vi "TestExec.Msg to Result, Float.vi"(8 "error in":errorcluster, 11 "Msg":string[](array[string])) -> (0 "error out":errorcluster, 3 "Result":T1)   [LabVIEW 2016]
uses:
  Controls/TestExec.Comparison Enum.ctl
  Controls/TestExec.Result Cluster, Float.ctl
panel:
  in  "Limits":variant
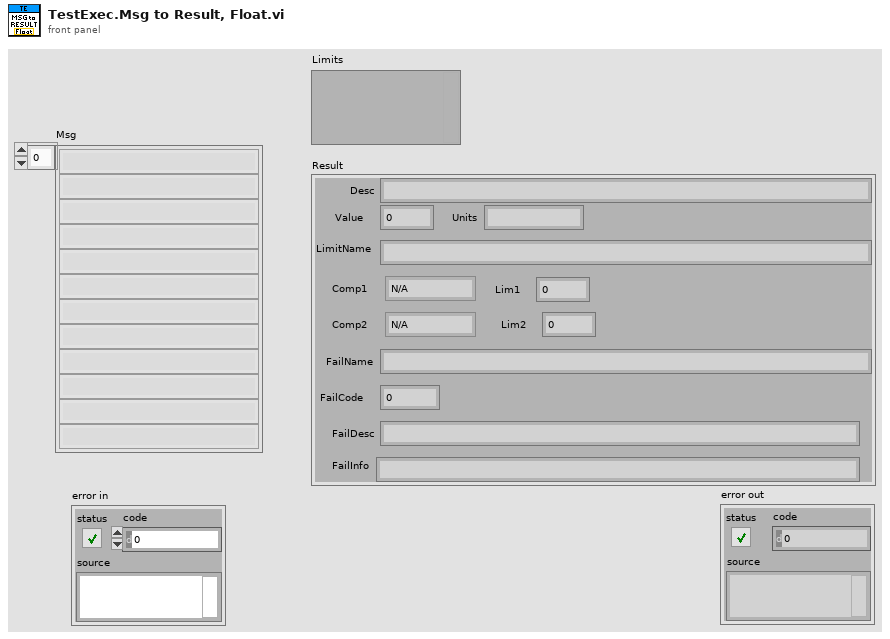
[diagram p1: front panel]
types:
  T1 = typedef "TestExec.Result Cluster, Float.ctl" = cluster{"Desc":string, "Value":dbl, "Units":string, "LimitName":string, "Comp1":T2, "Lim1":dbl, "Comp2":T2, "Lim2":dbl, "FailName":string, "FailCode":dbl, "FailDesc":string, "FailInfo":string}
  T2 = typedef "TestExec.Comparison Enum.ctl" = enum16{"N/A", "EQ", "NEQ", "LT", "LTE", "GT", "GTE"}
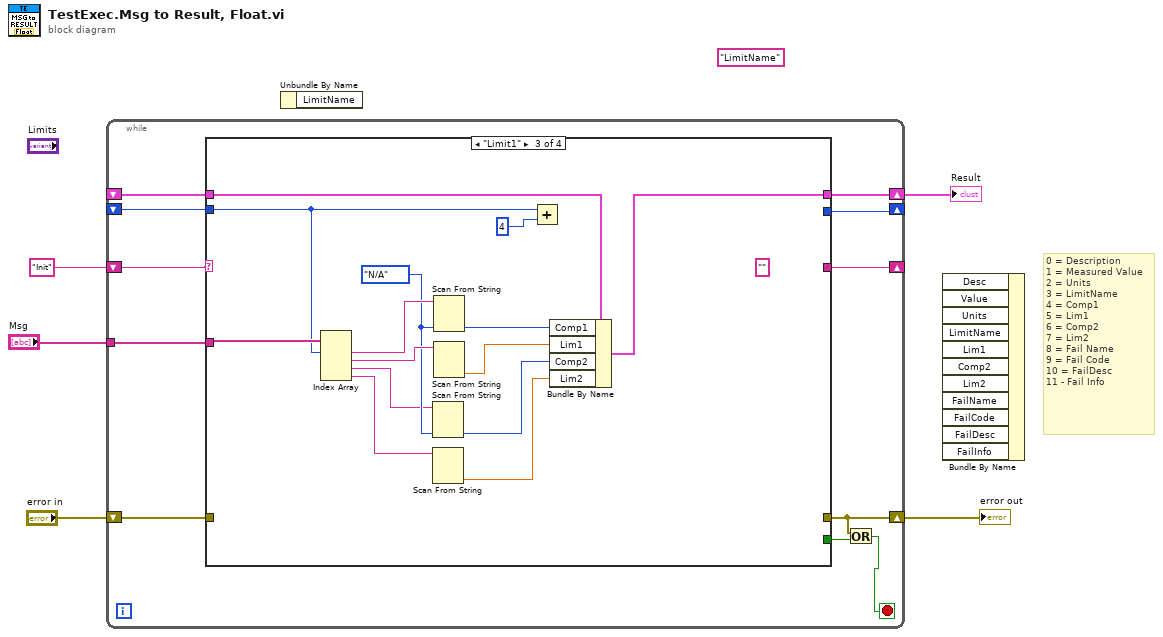
[diagram p0: block diagram]
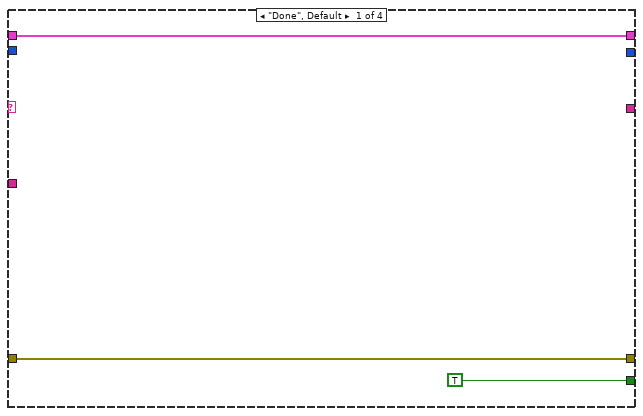
[diagram p2: hidden frame]
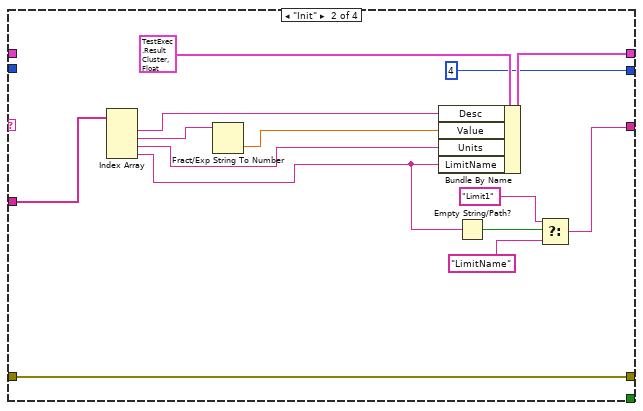
[diagram p3: hidden frame]
diagram:
  (unwired) "LimitName"
  # "0 = Description\t\n1 = Measured Value \n2 = Units\n3 = LimitName\t\n4 = Comp1\t\t\n5 = Lim1 \t\n6 = Comp2 \t\t\n7 = Lim2 \t\n8 = Fail Name\n9 = Fail Code\n10 = FailDesc\n11 - Fail Info"
  n1 = while {
    tunnel: "Msg" -> [w12]
    shift-right: [w13] -> _
    shift-left: "Init" -> [w14]
    shift-right: [w15] -> w3
    shift-left: _ -> [w16]
    shift-right: [w9] -> w1
    shift-left: "error in" -> [w11]
    shift-right: [w6] -> _
    shift-left: _ -> [w7]
    stop <- w8 stop-if-true
    n2 = case shown="\"Limit1\"" w14 {
      tunnel: w16 -> [w17 _ w47 _]
      tunnel: [w17 w32 w36 _] -> w15
      tunnel: [_ w23 _ _] -> w13
      tunnel: w12 -> [_ w31 w46 _]
      tunnel: w11 -> [w18 w26 _ _]
      tunnel: [w18 w26 _ _] -> w9
      tunnel: [TRUE _ _ _] -> w10
      tunnel: w7 -> [_ _ w35 _]
      tunnel: [_ 4 _ _] -> w6
      frame "Done", Default {
      }
      frame "Init" {
        n3 = Index Array(array=w31) -> (element #1=w30:string, element #2=w28:string, element #3=w27:string, element #4=w21:string)  [unwired: 4 in]
        n4 = Fract/Exp String To Number(string=w28) -> (number=w29:dbl)  [unwired: 3 in, 1 out]
        n5 = Bundle By Name(cluster=T1 {"Desc"="", "Value"=0.0, "Units"="", "LimitName"="", "Comp1"=enum."N/A", "Lim1"=0.0, "Comp2"=enum."N/A", "Lim2"=0.0, "FailName"="", "FailCode"=0.0, "FailDesc"="", "FailInfo"=""} ("Result"), "Desc"=w30, "Value"=w29, "Units"=w27, "LimitName"=w21) -> (w32:T1)
        n6 = Empty String/Path?(string/path=w21) -> (empty?=w20:bool)
        n7 = Select(t="Limit1", s=w20, f="LimitName") -> (s? t:f=w23:string)
      }
      frame "Limit1" {
        w39 = TestExec.Comparison_Enum."N/A" ("Comp1")
        (unwired) ""
        n8 = Index Array(array=w46, index #1=w35) -> (element #1=w45:string, element #2=w42:string, element #3=w38:string, element #4=w37:string)  [unwired: 3 in]
        n9 = Scan From String(input string=w38, default 1=w39) -> (output 1=w41:T2)  [unwired: 3 in, 3 out]
        n10 = Scan From String(input string=w37) -> (output 1=w40:dbl)  [unwired: 4 in, 3 out]
        n11 = Scan From String(input string=w45, default 1=w39) -> (output 1=w44:T2)  [unwired: 3 in, 3 out]
        n12 = Scan From String(input string=w42) -> (output 1=w43:dbl)  [unwired: 4 in, 3 out]
        n13 = Add(x=w35, y=4) -> ()  [unwired: 1 out]
        n14 = Bundle By Name(cluster=w47, "Comp1"=w44, "Lim1"=w43, "Comp2"=w41, "Lim2"=w40) -> (w36:T1)
      }
      frame "LimitName" {
      }
    }
    n15 = Or(x=w9, y=w10) -> (x .or. y?=w8:bool)
  }
  "error out" <- w1
  "Result" <- w3
  n16 = Unbundle By Name() -> ()  [unwired: 1 in, 1 out]
  n17 = Bundle By Name() -> ()  [unwired: 12 in, 1 out]
